vi "Configure OVP.vi"(6 "enabled (true)":bool=TRUE, 8 "error in (no error)":errorcluster, 9 "limit (0.0 Volts)":dbl[unit] format="%^.2e", 10 "channel name (\"CHANNEL1\")":string="CHANNEL1", 11 "CS++DCPwr in":refnum<class "CS++DCPwr.lvclass">) -> (0 "error out":errorcluster, 3 "CS++DCPwr out":refnum<class "CS++DCPwr.lvclass">)   [LabVIEW 2015, in "CS++DCPwr.lvlib" / "CS++DCPwr.lvclass"]
doc: "This VI configures the power supply's over-voltage protection. You specify the over-voltage limit and the behavior of the power supply when the output voltage is greater than or equal to that value.\n\nWhen the enabled parameter is FALSE, the limit parameter does not affect the instrument's behavior, and the driver ignores the limit parameter."
uses:
  CS++DCPwr.lvclass
  CSPP_Core/Classes/CS++ProcessVariables/ProcessVariable/PV.lvclass
  PV-Enum.ctl
  CSPP_Core/Classes/CS++ProcessVariables/ProcessVariable/PV.lvclass/PV.ctl
  CS++DCPwr.lvclass/CS++DCPwr.ctl
  CSPP_Core/Classes/CS++ProcessVariables/ProcessVariable/Write Data.vi
  CSPP_Core/Classes/CS++ProcessVariables/ProcessVariable/Write Timestamp.vi
  CSPP_Core/Classes/CS++ProcessVariables/ProcessVariable/Write Quality.vi
  CSPP_Core/Classes/CS++ProcessVariables/ProcessVariable/Write status.vi
  CSPP_Core/Classes/CS++ProcessVariables/PVConnection/PVConnection.lvclass
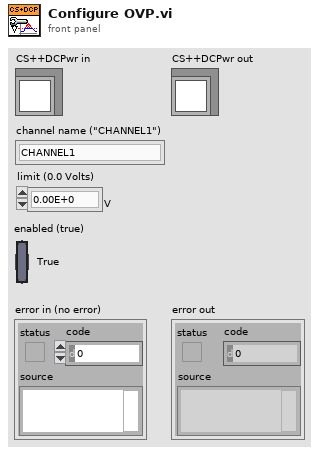
[diagram p1: front panel]
types:
  T1 = typedef "CS++DCPwr.lvlib/CS++DCPwr.lvclass/PV-Enum.ctl" = enum16{"CurrentLimit", "MaxCurrentLimit", "MaxVoltageLevel", "Measure-A", "Measure-V", "OVPLimit", "Range", "TriggerCurrentLimit", "TriggerVoltageLevel", "VoltageLevel", "Behavior", "DesiredOutputState", "RangeType", "TriggerSource", "InState", "OutputEnable", "OVPEnabled"}
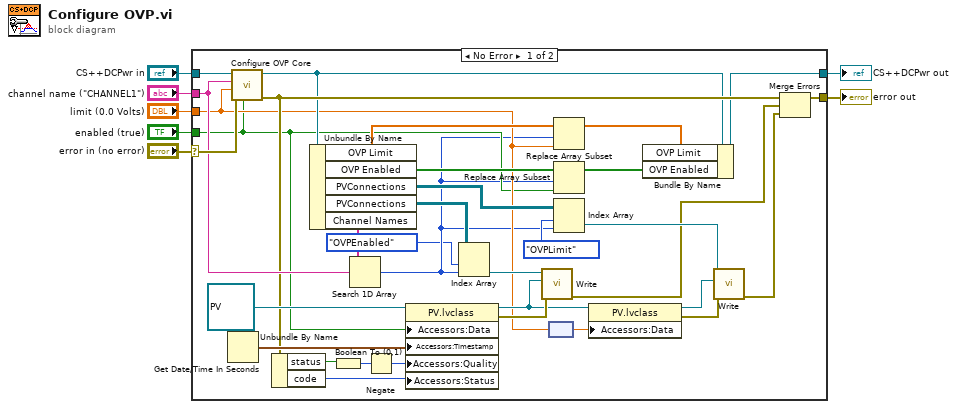
[diagram p0: block diagram]
diagram:
  n1 = case shown="No Error" "error in (no error)" {
    selector: "error in (no error)" -> [w40 w43]
    tunnel: [w32 w43] -> w1
    tunnel: [w23 w42] -> w2
    tunnel: "CS++DCPwr in" -> [w41 w42]
    tunnel: "channel name (\"CHANNEL1\")" -> [w35 _]
    tunnel: "enabled (true)" -> [w12 _]
    tunnel: "limit (0.0 Volts)" -> [w13 _]
    frame No Error {
      n2 = Get Date/Time In Seconds() -> (seconds since 1Jan1904=w39:timestamp)
      n3 = call-dynamic "Configure OVP Core.vi"("enabled (true)"=w12, "error in (no error)"=w40, "limit (0.0 Volts)"=w13, "channel name (\"CHANNEL1\")"=w35, "CS++DCPwr in"=w41) -> ("error out"=w27:errorcluster, "CS++DCPwr out"=w24:refnum<class "CS++DCPwr.lvclass">)  [unwired: 5 in]
      n4 = Unbundle By Name(w27) -> ("status"=w31:bool, "code"=w29:i32)
      n5 = Unbundle By Name(w24) -> ("OVP Limit"=w22:dbl[unit][], "OVP Enabled"=w26:bool[], "PVConnections"=w17:refnum<class "PVConnection.lvclass">[][], "PVConnections"=w34:refnum<class "PVConnection.lvclass">[][], "Channel Names"=w36:string[])
      n6 = Boolean To (0,1)(Boolean=w31) -> (0, 1=w30:i16)
      n7 = Search 1D Array(1D array=w36, element=w35) -> (index of element=w9:i32)  [unwired: 1 in]
      n8 = Negate(x=w30) -> (-x=w28:i16)
      n9 = property class="PV.lvclass"(reference=refnum<class "PV.lvclass"> refnum ("PV"), "Accessors:Data"=w12, "Accessors:Timestamp"=w39, "Accessors:Quality"=w28, "Accessors:Status"=w29) -> (reference out=w16:refnum<class "PV.lvclass">, error out=w37:errorcluster)  [unwired: 1 in]
      n10 = Index Array(array=w34, index (row)=PV-Enum."OVPEnabled" ("PV-Enum"), index (col)=w9) -> (element=w33:refnum<class "PVConnection.lvclass">)
      n11 = call "Write.vi"("error in (no error)"=w37, "PV"=w16, "PVConnection in"=w33) -> ("error out"=w15:errorcluster)  [unwired: 7 in, 1 out]
      n12 = node(w13) -> (w11:dbl)
      n13 = Replace Array Subset(array=w22, new element=w13, index=w9) -> (w21:dbl[unit][])
      n14 = Replace Array Subset(array=w26, new element=w12, index=w9) -> (w25:bool[])
      n15 = Index Array(array=w17, index (row)=PV-Enum."OVPLimit" ("PV-Enum"), index (col)=w9) -> (element=w20:refnum<class "PVConnection.lvclass">)
      n16 = property class="PV.lvclass"(reference=w16, "Accessors:Data"=w11) -> (reference out=w19:refnum<class "PV.lvclass">, error out=w18:errorcluster)  [unwired: 1 in]
      n17 = Bundle By Name(cluster=w24, "OVP Limit"=w21, "OVP Enabled"=w25) -> (w23:refnum<class "CS++DCPwr.lvclass">)
      n18 = call "Write.vi"("error in (no error)"=w18, "PV"=w19, "PVConnection in"=w20) -> ("error out"=w14:errorcluster)  [unwired: 7 in, 1 out]
      n19 = Merge Errors(w27, w15, w14) -> (w32:errorcluster)
    }
    frame Error {
    }
  }
  "error out" <- w1
  "CS++DCPwr out" <- w2
